vi "synth_set(SubVI).vi"(3 "dc offset?":bool=TRUE, 5 "dc offset":dbl, 6 "error in (no error)":errorcluster, 9 "VISA session":refnum<visa-resource-name>, 10 "amplitude (V)":ext=2.5, 11 "frequency (Hz)":ext=76.5) -> (2 "dup VISA session":refnum<visa-resource-name>, 4 "error out":errorcluster)   [LabVIEW 2014]
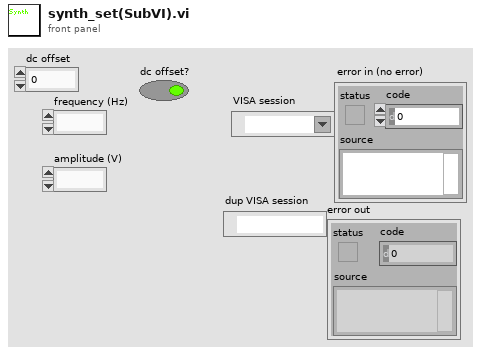
[diagram p1: front panel]
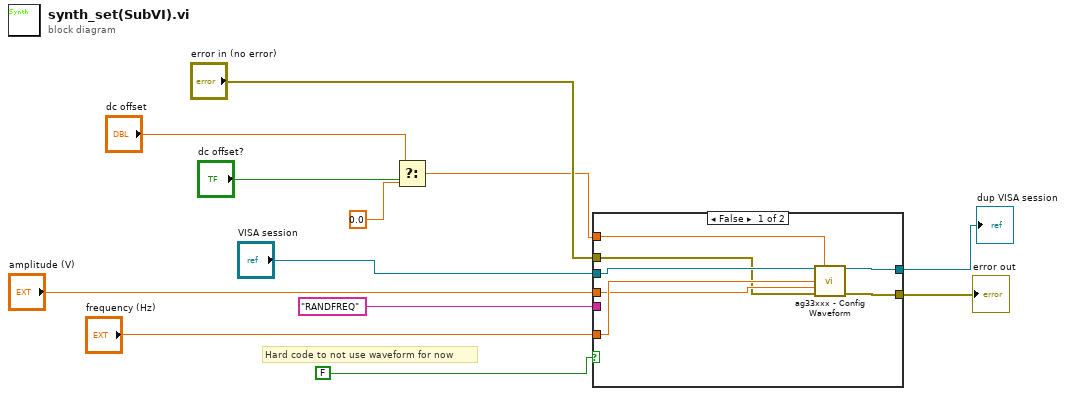
[diagram p0: block diagram]
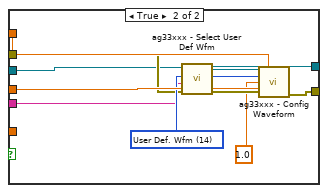
[diagram p2: hidden frame]
diagram:
  # "Hard code to not use waveform for now"
  n1 = Select(t="dc offset", s="dc offset?", f=0.0) -> (s? t:f=w8:dbl)
  n2 = case shown="False" FALSE ("chirp?") {
    tunnel: "VISA session" -> [w14 w24]
    tunnel: "error in (no error)" -> [w13 w25]
    tunnel: w8 -> [w19 w30]
    tunnel: "frequency (Hz)" -> [w18 _]
    tunnel: "amplitude (V)" -> [w17 w29]
    tunnel: [w16 w27] -> w5
    tunnel: [w15 w26] -> w4
    tunnel: "RANDFREQ" ("User Def. Wfm Name") -> [_ w21]
    frame False {
      n3 = call "ag33xxx - Config Waveform.vi"("VISA session"=w14, "Offset (0.00 V)"=w19, "Frequency (1000 Hz)"=w18, "Amplitude (0.1 Vpp)"=w17, "error in (no error)"=w13) -> ("dup VISA session"=w15:refnum<visa-resource-name>, "error out"=w16:errorcluster)  [unwired: 9 in]
    }
    frame True {
      w28 = u16 14 items=["DC"=0, "Sine"=1, "Square"=2, "Triangle"=3, "Ramp"=4, "Pulse"=6, "Noise"=7, "Sinc"=8, "Neg. Ramp"=9, "Exp. Rise"=10, "Exp. Fall"=11, "Cardiac"=12, "Volatile"=13, "User Def. Wfm"=14] ("Waveform Shape (1: Sine)")
      n4 = call "ag33xxx - Select User Def Wfm.vi"("error in (no error)"=w25, "User Def. Wfm Name"=w21, "VISA session"=w24) -> ("error out"=w22:errorcluster, "dup VISA session"=w23:refnum<visa-resource-name>)  [unwired: 7 in]
      n5 = call "ag33xxx - Config Waveform.vi"("VISA session"=w23, "Offset (0.00 V)"=w30, "Waveform Shape (1: Sine)"=w28, "Frequency (1000 Hz)"=1.0, "Amplitude (0.1 Vpp)"=w29, "error in (no error)"=w22) -> ("dup VISA session"=w26:refnum<visa-resource-name>, "error out"=w27:errorcluster)  [unwired: 8 in]
    }
  }
  "error out" <- w5
  "dup VISA session" <- w4
